vi "边缘检测+椭圆度.vi"(8 "error in (no error)":errorcluster, 10 "Image Dst":T1, 11 "Image Src":T1) -> (0 "error out":errorcluster, 1 "Ellipse":T2 {"Minor Axis"."Point 2"."Y" format="%.2f"; "Minor Axis"."Point 2"."X" format="%.2f"; "Minor Axis"."Point 1"."Y" format="%.2f"; "Minor Axis"."Point 1"."X" format="%.2f"; "Major Axis"."Point 2"."Y" format="%.2f"; "Major Axis"."Point 2"."X" format="%.2f"; "Major Axis"."Point 1"."Y" format="%.2f"; "Major Axis"."Point 1"."X" format="%.2f"; "Center"."Y" format="%.2f"; "Center"."X" format="%.2f"}, 2 "Image Out":T1, 3 "Particle Measurements (Pixels) (Particle Analysis 1)":dbl[][](array[numeric]) format="%.2f")   [LabVIEW 2015]
uses:
  <vilib>/vision/Image Controls.llb/IMAQ Image.ctl
  <vilib>/vision/NI_Vision_Development_Module.lvlib
panel:
  in  "Real-World Measurements (Particle Analysis 1)":i32[](array[ring]) items=["Center of Mass X", "Center of Mass Y", "First Pixel X", "First Pixel Y", "Bounding Rect Left", "Bounding Rect Top", "Bounding Rect Right", "Bounding Rect Bottom", "Max Feret Diameter Start X", "Max Feret Diameter Start Y", "Max Feret Diameter End X", "Max Feret Diameter End Y", "Max Horiz. Segment Length Left", "Max Horiz. Segment Length Right", "Max Horiz. Segment Length Row", "-", "Bounding Rect Width", "Bounding Rect Height", "Bounding Rect Diagonal", "Perimeter", "Convex Hull Perimeter", "Holes' Perimeter", "Max Feret Diameter", "Equivalent Ellipse Major Axis", "Equivalent Ellipse Minor Axis", "Equivalent Ellipse Minor Axis (Feret)", "Equivalent Rect Long Side", "Equivalent Rect Short Side", "Equivalent Rect Diagonal", "Equivalent Rect Short Side (Feret)", "Average Horiz. Segment Length", "Average Vert. Segment Length", "Hydraulic Radius", "Waddel Disk Diameter", "-", "Area", "Holes' Area", "Particle & Holes' Area", "Convex Hull Area", "Image Area", "-", "Number of Holes", "Number of Horiz. Segments", "Number of Vert. Segments", "-", "Orientation", "Max Feret Diameter Orientation", "-", "% Area/Image Area", "% Area/(Particle & Holes' Area)", "Ratio of Equivalent Ellipse Axes", "Ratio of Equivalent Rect Sides", "-", "Elongation Factor", "Compactness Factor", "Heywood Circularity Factor", "Type Factor", "-", "Sum X", "Sum Y", "Sum XX", "Sum XY", "Sum YY", "Sum XXX", "Sum XXY", "Sum XYY", "Sum YYY", "-", "Moment of Inertia XX", "Moment of Inertia XY", "Moment of Inertia YY", "Moment of Inertia XXX", "Moment of Inertia XXY", "Moment of Inertia XYY", "Moment of Inertia YYY", "Norm. Moment of Inertia XX", "Norm. Moment of Inertia XY", "Norm. Moment of Inertia YY", "Norm. Moment of Inertia XXX", "Norm. Moment of Inertia XXY", "Norm. Moment of Inertia XYY", "Norm. Moment of Inertia YYY", "Hu Moment 1", "Hu Moment 2", "Hu Moment 3", "Hu Moment 4", "Hu Moment 5", "Hu Moment 6", "Hu Moment 7"]
  in  "Pixel Measurements (Particle Analysis 1)":i32[](array[ring])=[0, 1] items=["Center of Mass X", "Center of Mass Y", "First Pixel X", "First Pixel Y", "Bounding Rect Left", "Bounding Rect Top", "Bounding Rect Right", "Bounding Rect Bottom", "Max Feret Diameter Start X", "Max Feret Diameter Start Y", "Max Feret Diameter End X", "Max Feret Diameter End Y", "Max Horiz. Segment Length Left", "Max Horiz. Segment Length Right", "Max Horiz. Segment Length Row", "-", "Bounding Rect Width", "Bounding Rect Height", "Bounding Rect Diagonal", "Perimeter", "Convex Hull Perimeter", "Holes' Perimeter", "Max Feret Diameter", "Equivalent Ellipse Major Axis", "Equivalent Ellipse Minor Axis", "Equivalent Ellipse Minor Axis (Feret)", "Equivalent Rect Long Side", "Equivalent Rect Short Side", "Equivalent Rect Diagonal", "Equivalent Rect Short Side (Feret)", "Average Horiz. Segment Length", "Average Vert. Segment Length", "Hydraulic Radius", "Waddel Disk Diameter", "-", "Area", "Holes' Area", "Particle & Holes' Area", "Convex Hull Area", "Image Area", "-", "Number of Holes", "Number of Horiz. Segments", "Number of Vert. Segments", "-", "Orientation", "Max Feret Diameter Orientation", "-", "% Area/Image Area", "% Area/(Particle & Holes' Area)", "Ratio of Equivalent Ellipse Axes", "Ratio of Equivalent Rect Sides", "-", "Elongation Factor", "Compactness Factor", "Heywood Circularity Factor", "Type Factor", "-", "Sum X", "Sum Y", "Sum XX", "Sum XY", "Sum YY", "Sum XXX", "Sum XXY", "Sum XYY", "Sum YYY", "-", "Moment of Inertia XX", "Moment of Inertia XY", "Moment of Inertia YY", "Moment of Inertia XXX", "Moment of Inertia XXY", "Moment of Inertia XYY", "Moment of Inertia YYY", "Norm. Moment of Inertia XX", "Norm. Moment of Inertia XY", "Norm. Moment of Inertia YY", "Norm. Moment of Inertia XXX", "Norm. Moment of Inertia XXY", "Norm. Moment of Inertia XYY", "Norm. Moment of Inertia YYY", "Hu Moment 1", "Hu Moment 2", "Hu Moment 3", "Hu Moment 4", "Hu Moment 5", "Hu Moment 6", "Hu Moment 7"]
  out "Particle Measurements (Real-World) (Particle Analysis 1)":dbl[][](array[numeric]) format="%.2f"
  out "Number of Particles (Particle Analysis 1)":i32
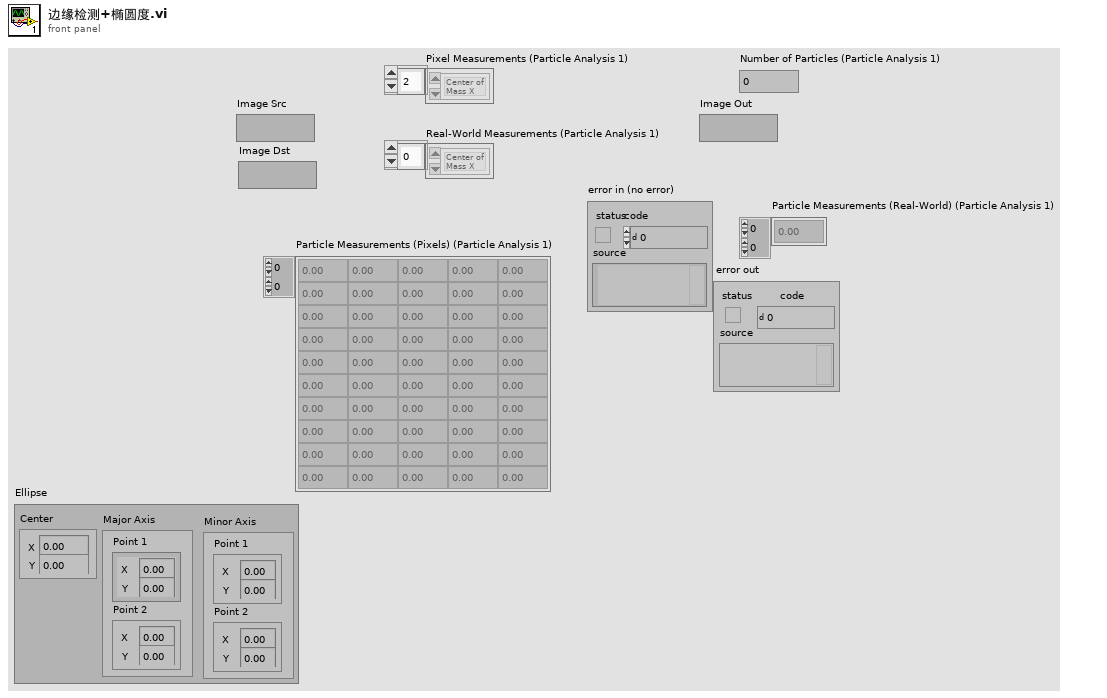
[diagram p1: front panel]
types:
  T1 = typedef "IMAQ Image.ctl" = refnum<image>
  T2 = cluster{"Center":cluster{"X":sgl, "Y":sgl}, "Major Axis":cluster{"Point 1":cluster{"X":sgl, "Y":sgl}, "Point 2":cluster{"X":sgl, "Y":sgl}}, "Minor Axis":cluster{"Point 1":cluster{"X":sgl, "Y":sgl}, "Point 2":cluster{"X":sgl, "Y":sgl}}}
  T3 = cluster{"Point 1":cluster{"X":sgl, "Y":sgl}, "Point 2":cluster{"X":sgl, "Y":sgl}}
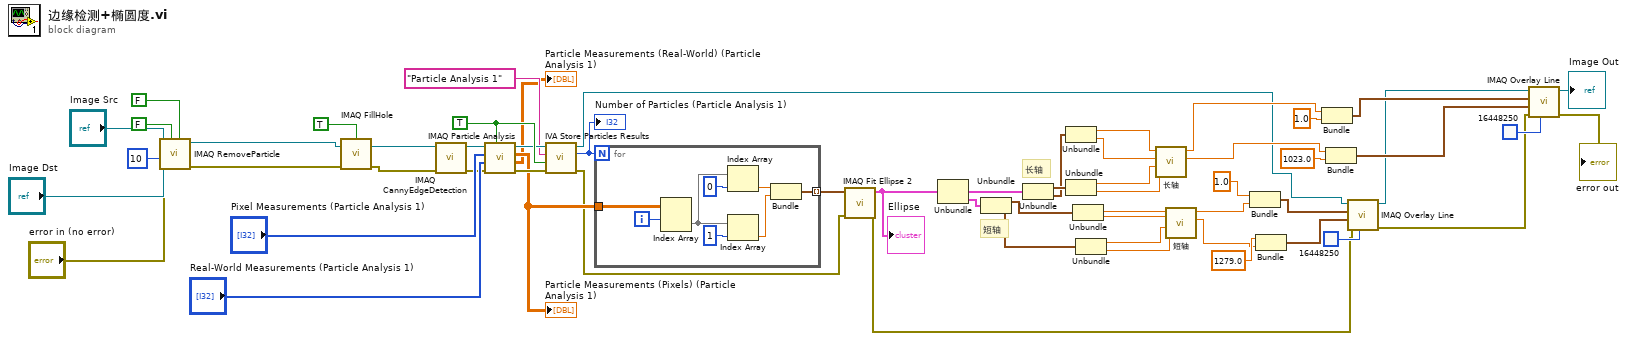
[diagram p0: block diagram]
diagram:
  w50 = TRUE ("Connectivity 4/8 (8)")
  # "长轴"
  # "短轴"
  n1 = call "IMAQ RemoveParticle"("Connectivity 4/8 (8)"=FALSE, "Square/Hexa (Square)"=FALSE, "error in (no error)"="error in (no error)", "Number of Erosion"=10, "Image Dst"="Image Dst", "Image Src"="Image Src") -> ("error out"=w56:errorcluster, "Image Dst Out"=w54:T1)  [unwired: 1 in, 3 out]
  n2 = call "IMAQ FillHole"("error in (no error)"=w56, "Image Src"=w54, "Connectivity 4/8 (8)"=TRUE) -> ("error out"=w27:errorcluster, "Image Dst Out"=w53:T1)  [unwired: 1 in, 2 out]
  n3 = call "IMAQ CannyEdgeDetection"("Image Src"=w53, "error in (no error)"=w27) -> ("Image Dst Out"=w41:T1, "error out"=w26:errorcluster)  [unwired: 6 in]
  n4 = call "IMAQ Particle Analysis"("Connectivity 4/8 (8)"=w50, "error in (no error)"=w26, "Real-World Measurements"="Real-World Measurements (Particle Analysis 1)", "Pixel Measurements"="Pixel Measurements (Particle Analysis 1)", "Image"=w41) -> ("error out"=w48:errorcluster, "Particle Measurements (Real-World)"=→"Particle Measurements (Real-World) (Particle Analysis 1)":dbl[][], "Particle Measurements (Pixels)"=w46:dbl[][], "Image Out (duplicate)"=w49:T1)  [unwired: 3 out]
  "Particle Measurements (Pixels) (Particle Analysis 1)" <- w46
  n5 = call <vilib>:"IVA Store Particles Results.vi"("error in (no error)"=w48, "Connectivity 4/8 (8)"=w50, "Step Name"="Particle Analysis 1", "Image in"=w49) -> ("error out"=w25:errorcluster, "Number of Particles"=w47:i32, "Image dup"=w11:T1)  [unwired: 5 out]
  "Number of Particles (Particle Analysis 1)" <- w47
  n6 = for {
    N: w47 -> [_]
    tunnel: w46 -> [w64]
    tunnel: [w65] -> w45 mode=indexing
    i -> [w63]
    n7 = Index Array(array=w64, index (row)=w63) -> (element=w62:dbl[])  [unwired: 1 in]
    n8 = Index Array(array=w62, index=0) -> (element=w61:dbl)
    n9 = Index Array(array=w62, index=1) -> (element=w60:dbl)
    n10 = Bundle("Numeric"=w61, "Numeric"=w60) -> (w65:cluster{"Numeric":dbl, "Numeric":dbl})  [unwired: 1 in]
  }
  n11 = call "IMAQ Fit Ellipse 2"("error in (no error)"=w25, "Radial Points"=w45) -> ("error out"=w8:errorcluster, "Ellipse"=w44:T2)  [unwired: 4 in, 4 out]
  "Ellipse" <- w44
  n12 = Unbundle(w44) -> ("Major Axis"=w43:T3, "Minor Axis"=w42:T3)  [unwired: 1 out]
  n13 = Unbundle(w42) -> ("Point 1"=w24:cluster{"X":sgl, "Y":sgl}, "Point 2"=w23:cluster{"X":sgl, "Y":sgl})
  n14 = Unbundle(w43) -> ("Point 1"=w40:cluster{"X":sgl, "Y":sgl}, "Point 2"=w39:cluster{"X":sgl, "Y":sgl})
  n15 = Unbundle(w39) -> ("X"=w35:sgl, "Y"=w34:sgl)
  n16 = Unbundle(w40) -> ("X"=w33:sgl, "Y"=w32:sgl)
  n17 = Unbundle(w24) -> ("X"=w22:sgl, "Y"=w21:sgl)
  n18 = Unbundle(w23) -> ("X"=w20:sgl, "Y"=w19:sgl)
  n19 = call "长轴.vi"("y2"=w32, "x2"=w33, "y1"=w34, "x1"=w35) -> ("第二点x值，y=479"=w30:dbl, "第一点x值，y=0"=w31:dbl)  [unwired: 5 in, 1 out]
  n20 = call "短轴.vi"("y2"=w19, "x2"=w20, "y1"=w21, "x1"=w22) -> ("第二点y值，x=639"=w14:dbl, "第一点y值，x=0"=w17:dbl)  [unwired: 5 in, 1 out]
  n21 = Bundle(1.0, "第一点y值，x=0"=w17) -> (w13:cluster{dbl, "第一点y值，x=0":dbl})  [unwired: 1 in]
  n22 = Bundle(1279.0, "第二点y值，x=639"=w14) -> (w12:cluster{dbl, "第二点y值，x=639":dbl})  [unwired: 1 in]
  n23 = Bundle("第一点x值，y=0"=w31, 1.0) -> (w29:cluster{"第一点x值，y=0":dbl, dbl})  [unwired: 1 in]
  n24 = Bundle("第二点x值，y=479"=w30, 1023.0) -> (w28:cluster{"第二点x值，y=479":dbl, dbl})  [unwired: 1 in]
  n25 = call "IMAQ Overlay Line"("Color"=u32 16448250, "error in (no error)"=w8, "End Point"=w12, "Start Point"=w13, "Image"=w11) -> ("error out"=w9:errorcluster, "Image Out"=w10:T1)  [unwired: 5 in]
  n26 = call "IMAQ Overlay Line"("Color"=u32 16448250, "error in (no error)"=w9, "End Point"=w28, "Start Point"=w29, "Image"=w10) -> ("error out"=→"error out":errorcluster, "Image Out"=→"Image Out":T1)  [unwired: 5 in]
